vi "Build.vi"(8 "error in (no error)":errorcluster, 11 "App-Builder":refnum<class "Builder.lvclass">) -> (0 "error out":errorcluster)   [LabVIEW 2025, in "App-Builder Library.lvlib" / "GUI Builder.lvclass"]
uses:
  GUI Builder.lvclass
  Builder/Builder.lvclass
  GUI Builder.lvclass/GUI Builder.ctl
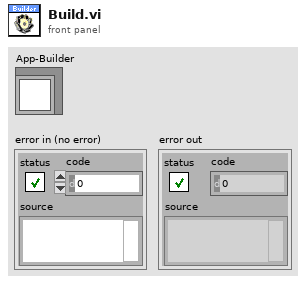
[diagram p1: front panel]
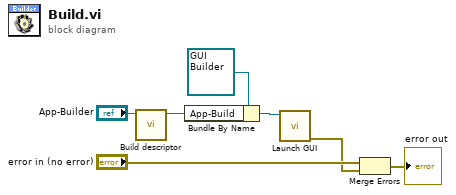
[diagram p0: block diagram]
diagram:
  n1 = call "Build descriptor.vi"("Builder in"="App-Builder") -> ("Builder out"=w2:refnum<class "Builder.lvclass">)  [unwired: 10 in]
  n2 = Bundle By Name(cluster=refnum<class "GUI Builder.lvclass"> refnum ("GUI Builder in"), "App-Build"=w2) -> (w3:refnum<class "GUI Builder.lvclass">)
  n3 = call "Launch GUI.vi"("GUI Builder in"=w3) -> ("error out"=w5:errorcluster)  [unwired: 10 in]
  n4 = Merge Errors("error in (no error)", w5) -> (→"error out":errorcluster)
